vi "ReadMoveListFile.vi"(1 "Application Directory":path, 2 "default name":path) -> (0 "Array":T1[](array[typedef]))   [LabVIEW 2017, in "RubikLibrary.lvlib"]
doc: "Read list of moves from preferences file:\n\nFile: <Application Folder>/preferences.txt\n\nMoves are enums from typedef \"SingmasterMoves\" i.e. U, L. DOes not handle ccw moves as U'."
uses:
  RubikLibrary.lvlib
  SingmasterMoves.ctl
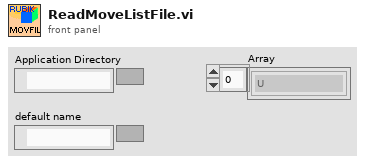
[diagram p1: front panel]
types:
  T1 = typedef "RubikLibrary.lvlib/SingmasterMoves.ctl" = enum16{"U", "L", "F", "R", "B", "D"}
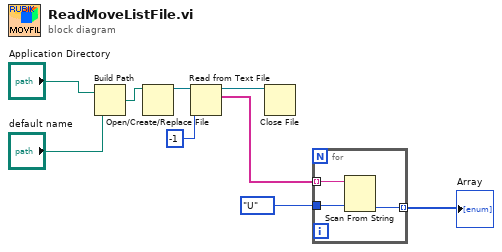
[diagram p0: block diagram]
diagram:
  n1 = Build Path(base path="Application Directory", name or relative path="default name") -> (appended path=w3:path)
  n2 = Open/Create/Replace File(file path (use dialog)=w3) -> (refnum out=w4:refnum<file>)  [unwired: 5 in, 2 out]
  n3 = Read from Text File(file (use dialog)=w4, count=-1) -> (refnum out=w6:refnum<file>, text=w9:string[])  [unwired: 2 in, 2 out]
  n4 = Close File(refnum=w6) -> ()  [unwired: 1 in, 2 out]
  n5 = for {
    tunnel: w9 -> [w12] mode=indexing
    tunnel: SingmasterMoves."U" ("Kociemba Moves") -> [w11]
    tunnel: [w10] -> w1 mode=indexing
    n6 = Scan From String(input string=w12, default 1=w11) -> (output 1=w10:T1)  [unwired: 3 in, 3 out]
  }
  "Array" <- w1
